vi "FVIR_Setup_Selection.vi"(6 "Select test case":i32(listbox), 8 "error in (no error)":errorcluster, 11 "UI in":refnum<queue>) -> (0 "error out":errorcluster, 3 "UI out":refnum<queue>, 4 "Test Case - FVIR":string)   [LabVIEW 2020]
uses:
  Message Queue/Message Cluster.ctl
  Message Queue/Enqueue Message (Single).vi
  Message Queue/Message Queue.lvlib
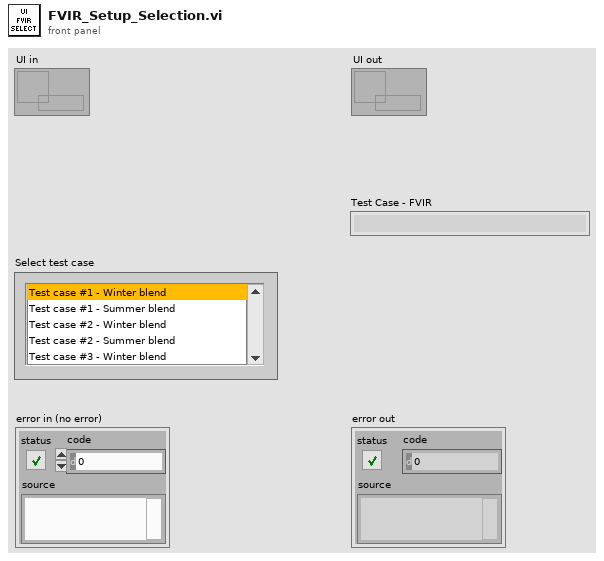
[diagram p1: front panel]
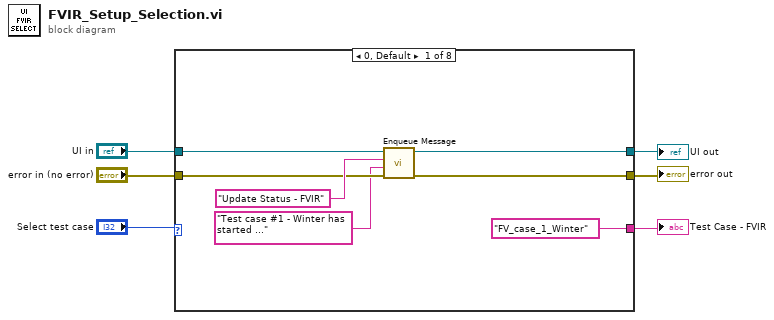
[diagram p0: block diagram]
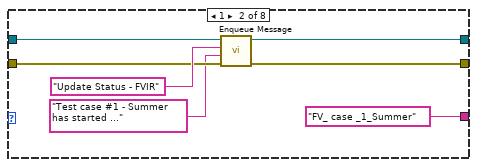
[diagram p2: hidden frame]
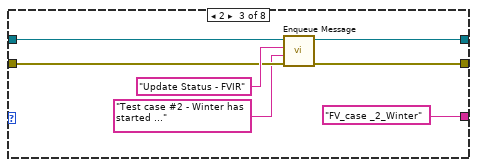
[diagram p3: hidden frame]
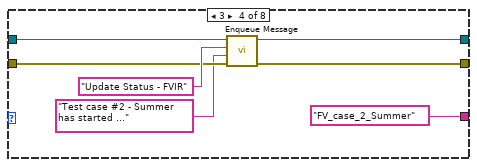
[diagram p4: hidden frame]
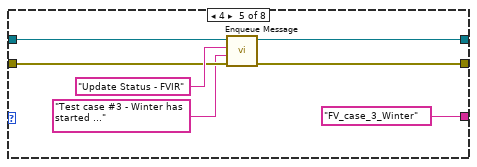
[diagram p5: hidden frame]
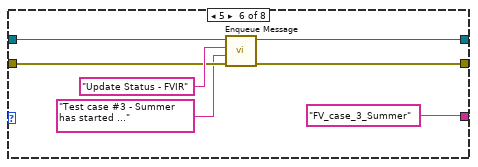
[diagram p6: hidden frame]
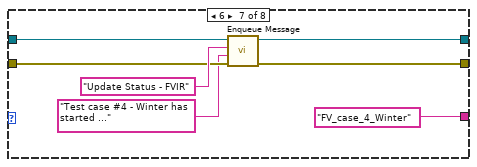
[diagram p7: hidden frame]
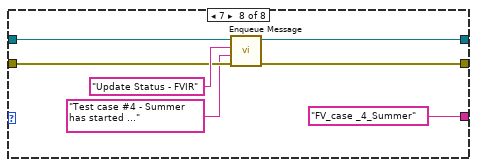
[diagram p8: hidden frame]
diagram:
  n1 = case shown="0, Default" "Select test case" {
    tunnel: "UI in" -> [w12 w19 w26 w33 w40 w47 w54 w61]
    tunnel: "error in (no error)" -> [w11 w18 w25 w32 w39 w46 w53 w60]
    tunnel: ["FV_case_1_Winter" ("Acquiring and Logging...") "FV_ case _1_Summer" ("Acquiring and Logging...") "FV_case _2_Winter" ("Acquiring and Logging...") "FV_case_2_Summer" ("Acquiring and Logging...") "FV_case_3_Winter" ("Acquiring and Logging...") "FV_case_3_Summer" ("Acquiring and Logging...") "FV_case_4_Winter" ("Acquiring and Logging...") "FV_case _4_Summer" ("Acquiring and Logging...")] -> w4
    tunnel: [w8 w15 w22 w29 w36 w43 w50 w57] -> w5
    tunnel: [w7 w14 w21 w28 w35 w42 w49 w56] -> w2
    frame 0, Default {
      n2 = call-poly "Enqueue Message.vi"("error in (no error)"=w11, "Message Data"="Test case #1 - Winter has started ..." ("Acquiring and Logging..."), "Message"="Update Status - FVIR", "Message Queue"=w12) -> ("error out"=w7:errorcluster, "dup Message Queue"=w8:refnum<queue>)  [unwired: 6 in]
    }
    frame 1 {
      n3 = call-poly "Enqueue Message.vi"("error in (no error)"=w18, "Message Data"="Test case #1 - Summer has started ..." ("Acquiring and Logging..."), "Message"="Update Status - FVIR", "Message Queue"=w19) -> ("error out"=w14:errorcluster, "dup Message Queue"=w15:refnum<queue>)  [unwired: 6 in]
    }
    frame 2 {
      n4 = call-poly "Enqueue Message.vi"("error in (no error)"=w25, "Message Data"="Test case #2 - Winter has started ..." ("Acquiring and Logging..."), "Message"="Update Status - FVIR", "Message Queue"=w26) -> ("error out"=w21:errorcluster, "dup Message Queue"=w22:refnum<queue>)  [unwired: 6 in]
    }
    frame 3 {
      n5 = call-poly "Enqueue Message.vi"("error in (no error)"=w32, "Message Data"="Test case #2 - Summer has started ..." ("Acquiring and Logging..."), "Message"="Update Status - FVIR", "Message Queue"=w33) -> ("error out"=w28:errorcluster, "dup Message Queue"=w29:refnum<queue>)  [unwired: 6 in]
    }
    frame 4 {
      n6 = call-poly "Enqueue Message.vi"("error in (no error)"=w39, "Message Data"="Test case #3 - Winter has started ..." ("Acquiring and Logging..."), "Message"="Update Status - FVIR", "Message Queue"=w40) -> ("error out"=w35:errorcluster, "dup Message Queue"=w36:refnum<queue>)  [unwired: 6 in]
    }
    frame 5 {
      n7 = call-poly "Enqueue Message.vi"("error in (no error)"=w46, "Message Data"="Test case #3 - Summer has started ..." ("Acquiring and Logging..."), "Message"="Update Status - FVIR", "Message Queue"=w47) -> ("error out"=w42:errorcluster, "dup Message Queue"=w43:refnum<queue>)  [unwired: 6 in]
    }
    frame 6 {
      n8 = call-poly "Enqueue Message.vi"("error in (no error)"=w53, "Message Data"="Test case #4 - Winter has started ..." ("Acquiring and Logging..."), "Message"="Update Status - FVIR", "Message Queue"=w54) -> ("error out"=w49:errorcluster, "dup Message Queue"=w50:refnum<queue>)  [unwired: 6 in]
    }
    frame 7 {
      n9 = call-poly "Enqueue Message.vi"("error in (no error)"=w60, "Message Data"="Test case #4 - Summer has started ..." ("Acquiring and Logging..."), "Message"="Update Status - FVIR", "Message Queue"=w61) -> ("error out"=w56:errorcluster, "dup Message Queue"=w57:refnum<queue>)  [unwired: 6 in]
    }
  }
  "error out" <- w2
  "UI out" <- w5
  "Test Case - FVIR" <- w4
